vi "raptor_end_scan.vi"(8 "error in (no error)":errorcluster) -> (0 "error out":errorcluster)   [LabVIEW 2016]
doc: "Raptor: Stops the current scan,"
uses:
  typedef/raptor_message.ctl
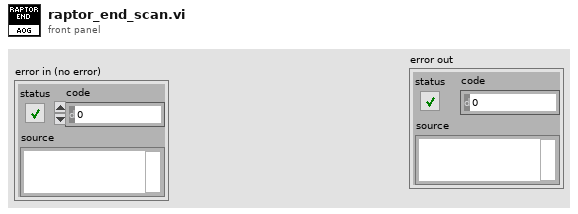
[diagram p1: front panel]
types:
  T1 = typedef "raptor_message.ctl" = cluster{"Message":enum16{"start", "stop", "initialise", "shutdown", "end scan", "new scan", "set depth"}, "Data":variant}
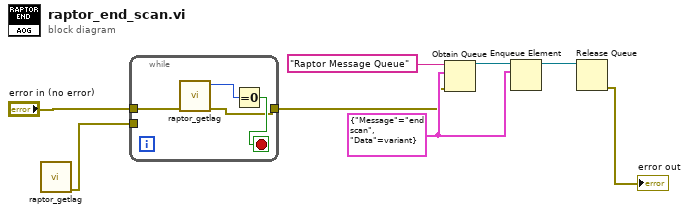
[diagram p0: block diagram]
diagram:
  w6 = T1 {"Message"=enum."end scan", "Data"=variant} ("Cluster")
  n1 = call "raptor_getlag.vi"() -> ("error out"=w1:errorcluster)  [unwired: 10 in, 1 out]
  n2 = while {
    tunnel: [w10] -> w3
    tunnel: "error in (no error)" -> [w9]
    tunnel: w1 -> [_]
    stop <- w11 stop-if-true
    n3 = call "raptor_getlag.vi"("error in (no error)"=w9) -> ("error out"=w10:errorcluster, "Frame Lag"=w12:i32)  [unwired: 9 in]
    n4 = Equal To 0?(x=w12) -> (x = 0?=w11:bool)
  }
  n5 = Obtain Queue(name (unnamed)="Raptor Message Queue", element data type=w6, error in (no error)=w3) -> (queue out=w7:refnum<queue>)  [unwired: 2 in, 2 out]
  n6 = Enqueue Element(queue=w7, element=w6) -> (queue out=w5:refnum<queue>)  [unwired: 2 in, 2 out]
  n7 = Release Queue(queue=w5) -> (error out=→"error out":errorcluster)  [unwired: 2 in, 2 out]
